vi "Key and Mouse Monitor.vi"() -> ()   [LabVIEW 2013, in "Multiple LV2 Global.lvlib"]
uses:
  Multiple LV2 Global.lvlib
  LV Config Write String.vi
  LV Config Read String.vi
panel:
  out "Mouse Pos":string
  out "Pic":picture
  in  "停止":bool
  out "Key Pressed":string
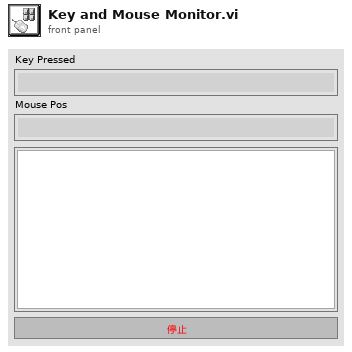
[diagram p1: front panel]
types:
  T1 = typedef "LVPoint32TypeDef.ctl" = cluster{"Horizontal":i32, "Vertical":i32}
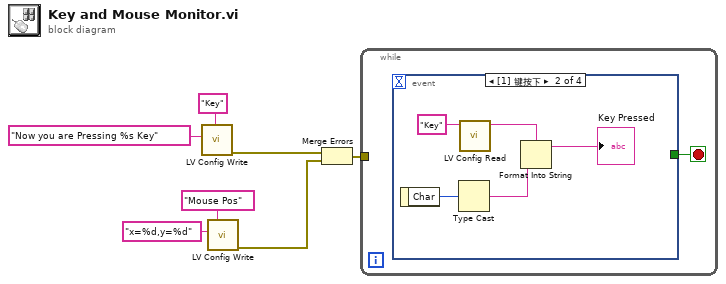
[diagram p0: block diagram]
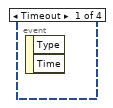
[diagram p2: hidden frame]
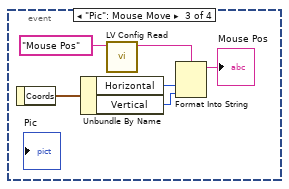
[diagram p3: hidden frame]
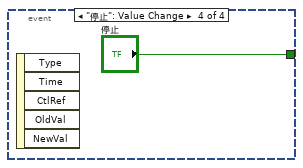
[diagram p4: hidden frame]
diagram:
  n1 = call-poly "LV Config Write.vi"("value"="Now you are Pressing %s Key", "key"="Key") -> ("error out"=w3:errorcluster)  [unwired: 5 in]
  n2 = call-poly "LV Config Write.vi"("value"="x=%d,y=%d", "key"="Mouse Pos") -> ("error out"=w2:errorcluster)  [unwired: 5 in]
  n3 = Merge Errors(w3, w2) -> (w1:errorcluster)
  n4 = while {
    tunnel: w1 -> [_]
    stop <- w8 stop-if-true
    n5 = event shown="[1] 键按下" {
      selector: _ -> [_ _ _ _]
      dyn-events: _ -> [_ _ _ _]
      timeout: _ -> [_ _ _ _]
      tunnel: [_ _ _ "停止"] -> w8
      event Timeout {
        n6 = event-data() -> ()  [unwired: 1 in, 2 out]
      }
      event Key Down {
        n7 = event-data() -> ("Char"=w13:i16)  [unwired: 1 in]
        n8 = Type Cast(x=w13) -> (*(type *) &x=w10:string)  [unwired: 1 in]
        n9 = call-poly "LV Config Read.vi"("key"="Key") -> ("value"=w11:string)  [unwired: 4 in, 2 out]
        n10 = Format Into String(format string=w11, w10) -> (resulting string=→"Key Pressed":string)  [unwired: 2 in, 1 out]
      }
      event "Pic": Mouse Move {
        n11 = event-data() -> ("Coords"=w19:T1)  [unwired: 1 in]
        n12 = Unbundle By Name(w19) -> ("Horizontal"=w17:i32, "Vertical"=w16:i32)
        n13 = call-poly "LV Config Read.vi"("key"="Mouse Pos" ("default value")) -> ("value"=w18:string)  [unwired: 4 in, 2 out]
        n14 = Format Into String(format string=w18, w17, w16) -> (resulting string=→"Mouse Pos":string)  [unwired: 2 in, 1 out]
      }
      event "停止": Value Change {
        n15 = event-data() -> ()  [unwired: 1 in, 5 out]
      }
    }
  }
